vi "muPathSamplingFPGA27.vi"() -> ()   [LabVIEW 2017]
uses:
  <vilib>/rvi/Emulation/niFpgaSctlEmulationGetInTimedLoop.vi
  <vilib>/rvi/Emulation/niFpgaProcessEmulError.vi
  <vilib>/rvi/Emulation/niFpgaGetClockAttributes.vi
  <vilib>/rvi/Emulation/niFpgaEmulationReportErrorSimple.vi
  <vilib>/rvi/eio/common/nirviEmuTemplateMethod_errors.vi
  <vilib>/rvi/Emulation/niFpgaCriticalErrorInLSC.vi
  <vilib>/rvi/interface/RandomDataEmulation/niFpgaRandomDataHandleErrors.vi
  <vilib>/eio/EIONode/EIONode.xnode
  <vilib>/rvi/DataTransferAndStorage/Container/XNode/niFpgaContainer.xnode
  <vilib>/rvi/interface/RandomDataEmulation/nirviRandomDataFpgaReadWriteTemplate.vi
panel:
  in  "pixel segment":u32
  out "x output":fxp<+/-,64,29>=0.00029289722442626953
  out "x sensor":fxp<+/-,20,5>
  out "y output":fxp<+/-,64,29>=0.29396580904722214
  out "y sensor":fxp<+/-,20,5>=-0.285125732421875
  in  "XY Clock (uSec)":fxp<+,32,32>=50.0
  out "z output":fxp<+/-,64,29>=-3.5890110712498426
  out "deflection sensor":fxp<+/-,20,5>=-0.271331787109375
  in  "Z Clock (uSec)":fxp<+,32,32>=10.0
  out "ToRead":u32
  in  "Stage Clock (uSec)":fxp<+,32,32>=500.0
  in  "Sampling Clock (uSec)":fxp<+,32,32>=1500.0
  in  "muPathUpdate Clock (uSec)":fxp<+,32,32>=2400.0
  in  "initial image_x":u16=1
  in  "initial image_y":u16=1
  out "zControlMode":bool
  out "a tor buffer":fxp<+,17,1>[](array[numeric])=[1.9999847412109375, 1.9999847412109375, 1.9999847412109375, 1.9999847412109375, 1.9999847412109375, 1.9999847412109375, 1.9999847412109375, 1.9999847412109375, 1.9999847412109375, 1.9999847412109375, 1.9999847412109375, 1.9999847412109375, 1.9999847412109375, 1.9999847412109375, 1.9999847412109375, 1.9999847412109375, 1.9999847412109375, 1.9999847412109375, 1.9999847412109375, 1.9999847412109375, 1.9999847412109375, 1.9999847412109375, 1.9999847412109375, 1.9999847412109375, 1.9999847412109375]
  out "b tor buffer":fxp<+,17,1>[](array[numeric])=[1.9999847412109375, 1.9999847412109375, 1.9999847412109375, 1.9999847412109375, 1.9999847412109375, 1.9999847412109375, 1.9999847412109375, 1.9999847412109375, 1.9999847412109375, 1.9999847412109375, 1.9999847412109375, 1.9999847412109375, 1.9999847412109375, 1.9999847412109375, 1.9999847412109375, 1.9999847412109375, 1.9999847412109375, 1.9999847412109375, 1.9999847412109375, 1.9999847412109375, 1.9999847412109375, 1.9999847412109375, 1.9999847412109375, 1.9999847412109375, 1.9999847412109375]
  out "x_pos":fxp<+/-,50,5>=0.005859375
  out "y_pos":fxp<+/-,50,5>=0.005859375
  out "signalToStop":bool
  in  "deflection control":T1={"SetPoint (V)"=0.0, "scanning I"=0.03125, "scanning P"=0.0498046875, "Initial I (V)"=0.0, "Upper Limit (V)"=8.0, "Lower Limit (V)"=-8.0, "approach I"=0.03125, "approach P"=0.0498046875}
  in  "z control":T2={"SetPoint (V)"=-0.19999980926513672, "I"=0.03125, "P"=0.0498046875, "Initial I (V)"=0.0, "Upper Limit (V)"=8.0, "Lower Limit (V)"=-8.0}
  out "stageIndicator":u8=1
  in  "x threshold":fxp<+/-,20,5>=0.0050048828125
  in  "y threshold":fxp<+/-,20,5>=0.0050048828125
  in  "z threshold":fxp<+/-,20,5>=0.0050048828125
  in  "deflection threshold":fxp<+/-,20,5>=0.0050048828125
  out "length":u16
  out "direction":u16
  out "x_FinalPos":fxp<+/-,50,5>
  out "y_FinalPos":fxp<+/-,50,5>
  out "SettleCheckBuffer":u16=25
  in  "y control":T3={"SetPoint (V)"=0.0, "scanning I"=0.03125, "scanning P"=0.0498046875, "Initial I (V)"=0.0, "Upper Limit (V)"=8.0, "Lower Limit (V)"=-8.0, "move I"=0.03125, "move P"=0.0302734375}
  in  "x control":T3={"SetPoint (V)"=0.0, "scanning I"=0.03125, "scanning P"=0.0498046875, "Initial I (V)"=0.0, "Upper Limit (V)"=8.0, "Lower Limit (V)"=-8.0, "move I"=0.03125, "move P"=0.0498046875}
  out "signalToInitialStageStop":bool
  out "mupathfinishSignal":bool
  in  "ImageToSample":T4={"image size_x"=256, "image size_y"=256, "sample start_x"=0.0, "sample start_y"=0.0, "sample end_x"=3.0, "sample end_y"=3.0}
  out "increment_x":fxp<+/-,50,5>=0.01171875
  out "increment_y":fxp<+/-,50,5>=0.01171875
  out "x_image_pos":u16
  out "y_image_pos":u16
  in  "x_scan threshold":fxp<+/-,20,5>=0.0050048828125
  in  "y_scan threshold":fxp<+/-,20,5>=0.0050048828125
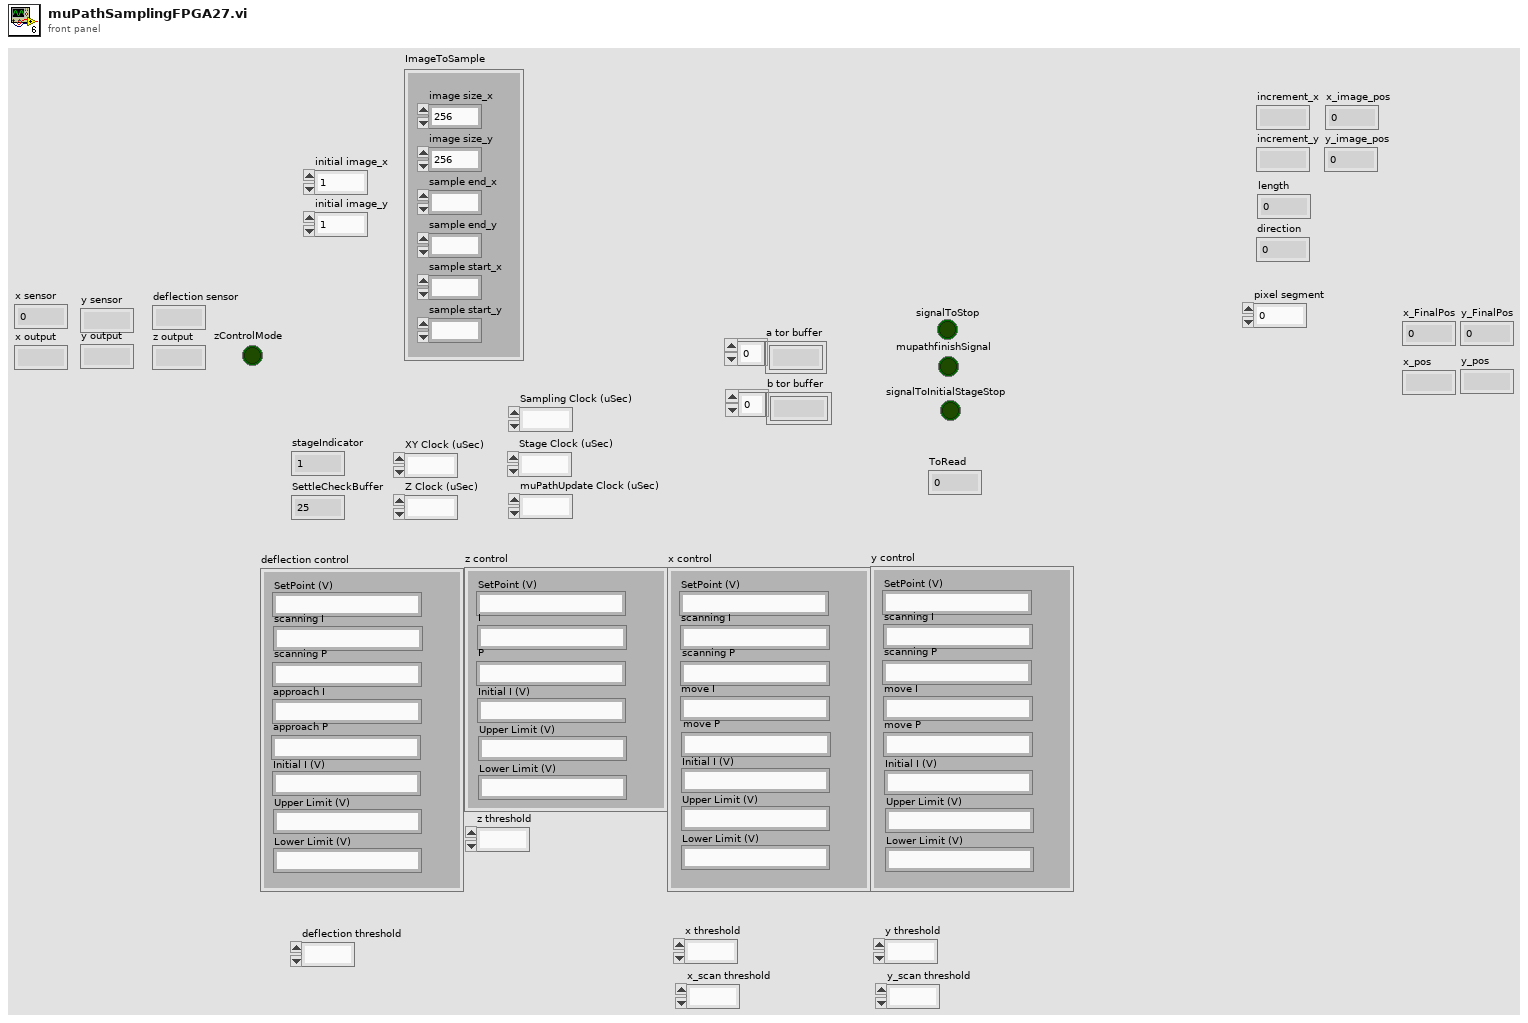
[diagram p1: front panel]
types:
  T1 = cluster{"SetPoint (V)":fxp<+/-,26,5>, "scanning I":fxp<+,21,13>, "scanning P":fxp<+,15,5>, "Initial I (V)":fxp<+/-,10,5>, "Upper Limit (V)":fxp<+/-,26,5>, "Lower Limit (V)":fxp<+/-,26,5>, "approach I":fxp<+,21,13>, "approach P":fxp<+,15,5>}
  T2 = cluster{"SetPoint (V)":fxp<+/-,26,5>, "I":fxp<+,21,13>, "P":fxp<+,15,5>, "Initial I (V)":fxp<+/-,10,5>, "Upper Limit (V)":fxp<+/-,26,5>, "Lower Limit (V)":fxp<+/-,26,5>}
  T3 = cluster{"SetPoint (V)":fxp<+/-,26,5>, "scanning I":fxp<+,21,13>, "scanning P":fxp<+,15,5>, "Initial I (V)":fxp<+/-,10,5>, "Upper Limit (V)":fxp<+/-,26,5>, "Lower Limit (V)":fxp<+/-,26,5>, "move I":fxp<+,21,13>, "move P":fxp<+,15,5>}
  T4 = cluster{"image size_x":u16, "image size_y":u16, "sample start_x":fxp<+/-,26,5>, "sample start_y":fxp<+/-,26,5>, "sample end_x":fxp<+/-,26,5>, "sample end_y":fxp<+/-,26,5>}
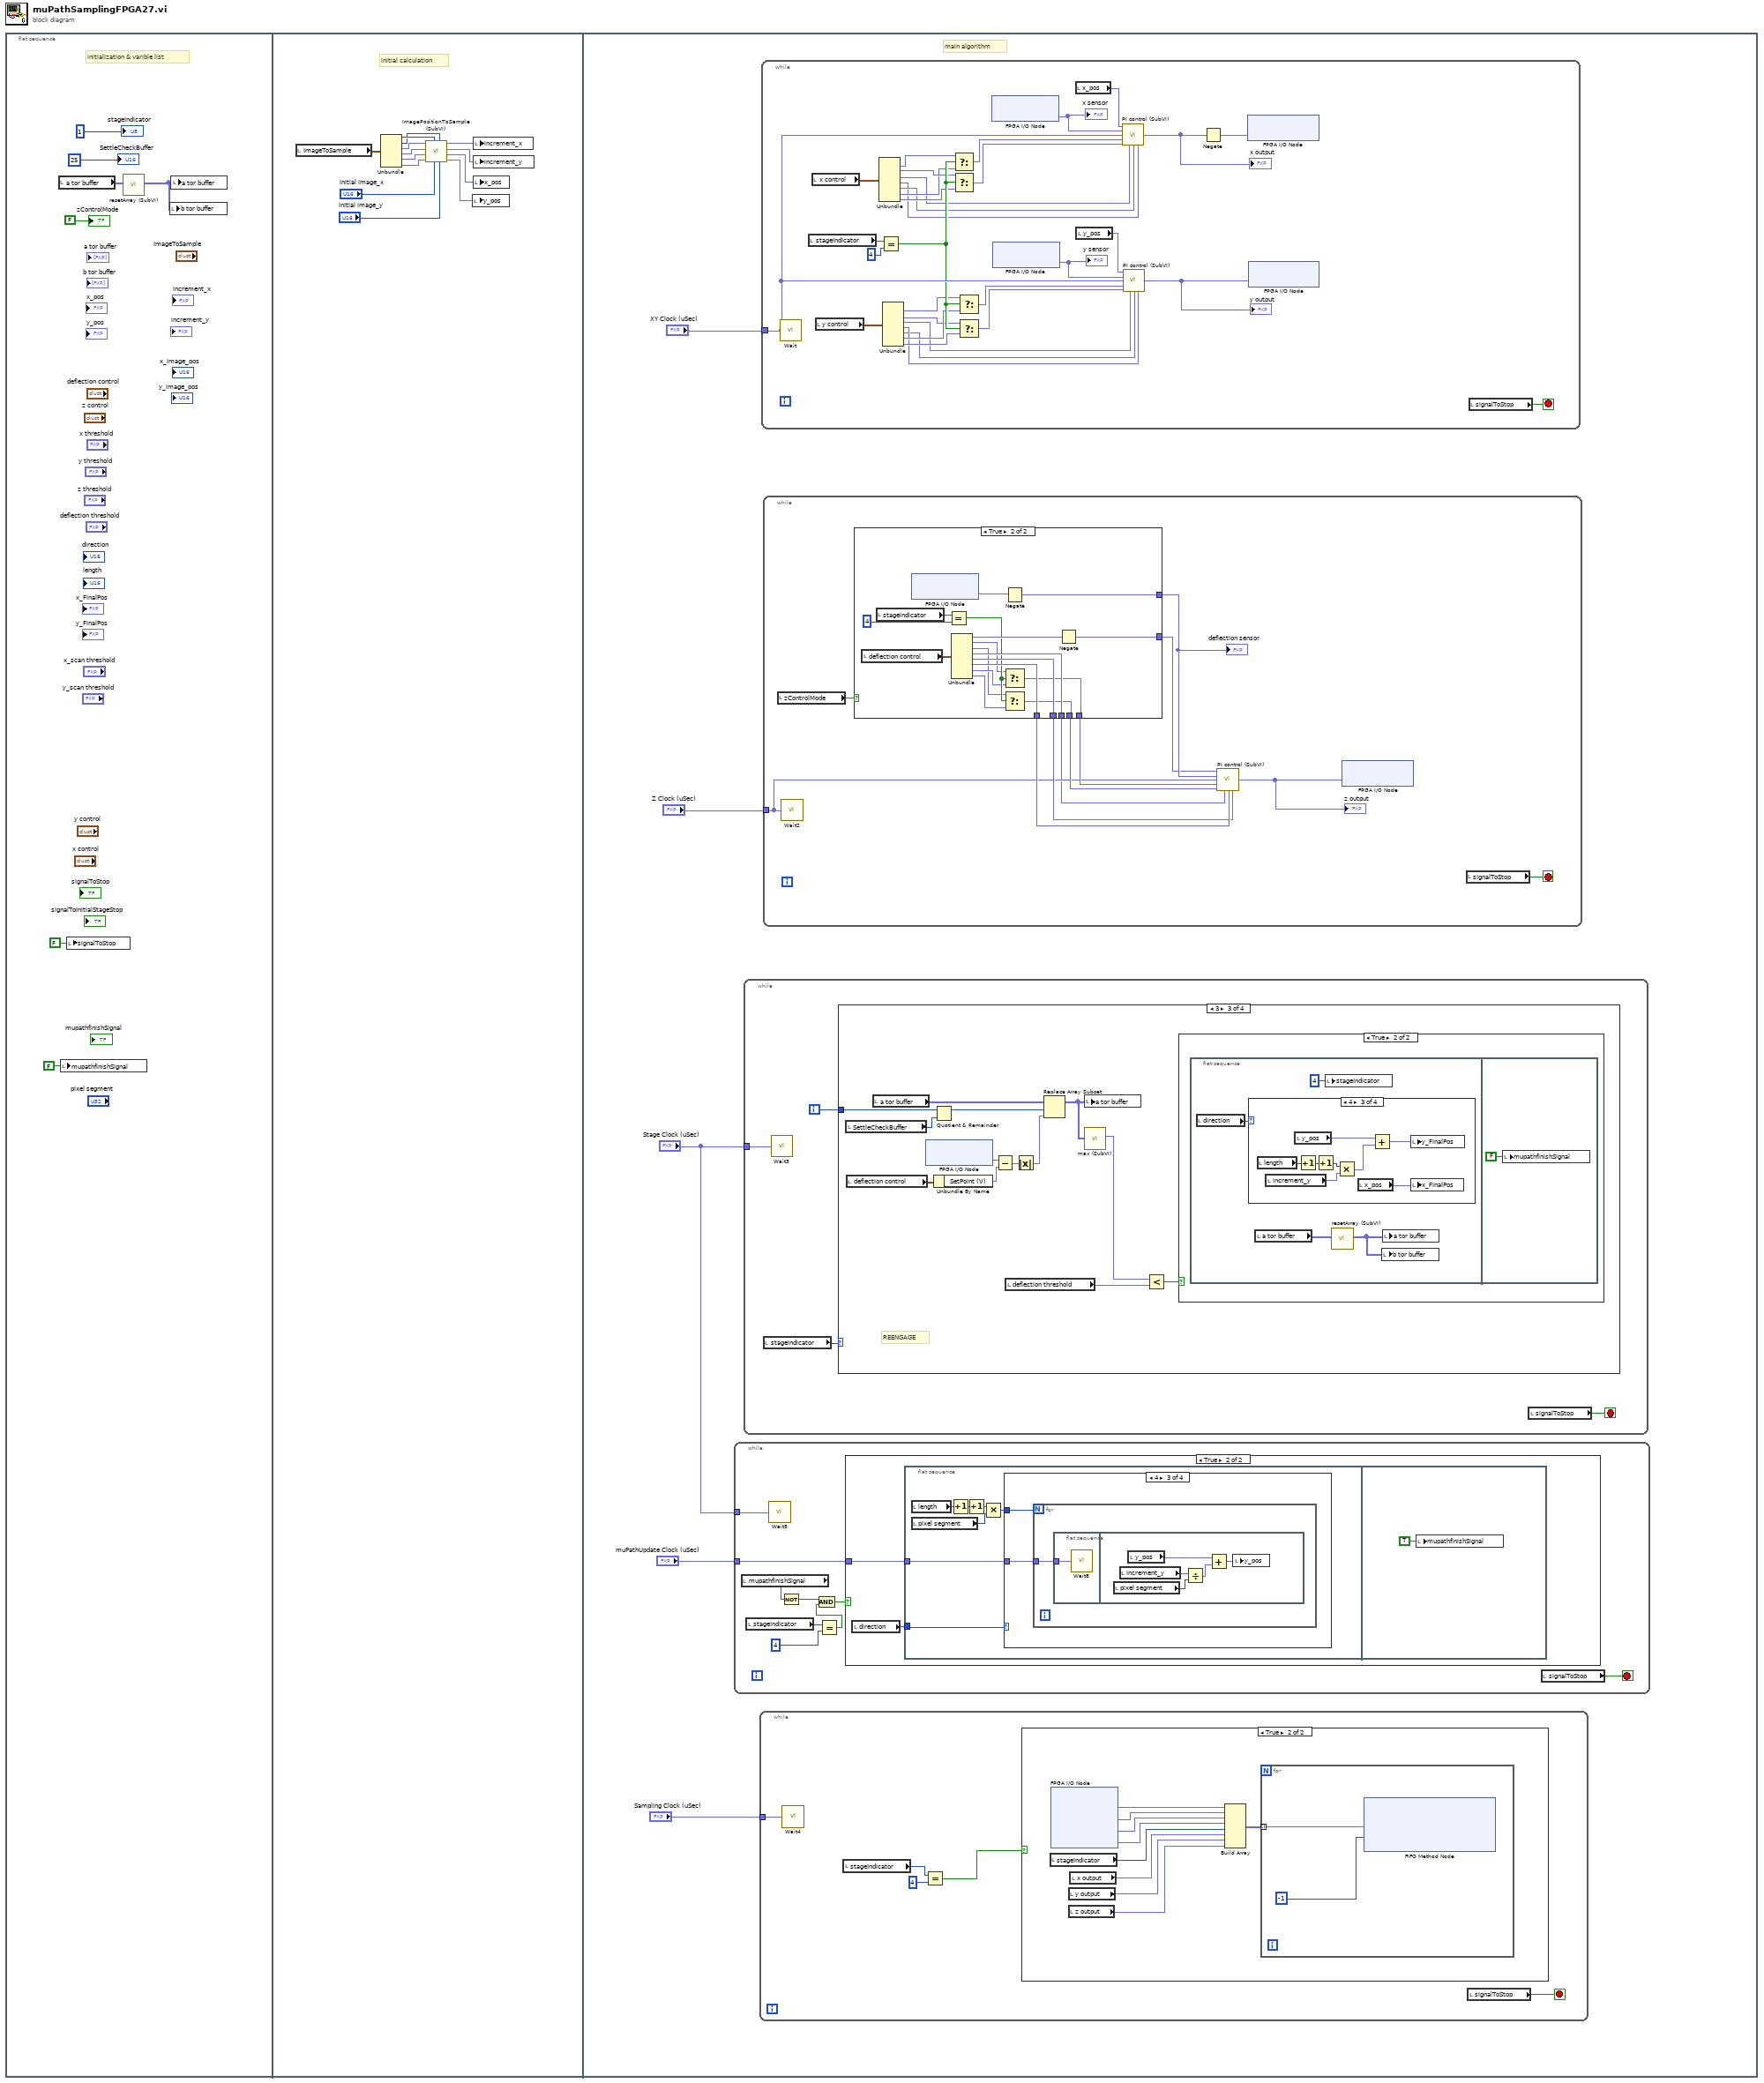
[diagram p0: block diagram]
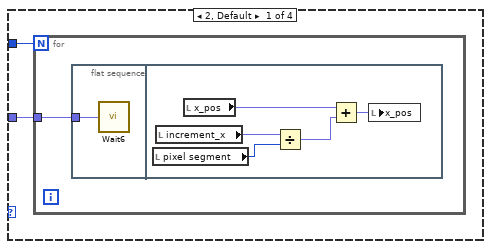
[diagram p3: hidden frame]
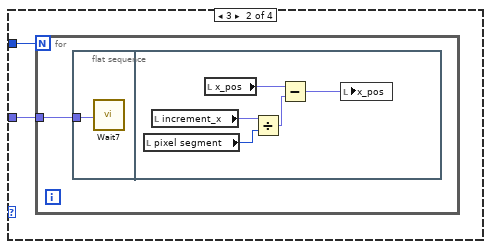
[diagram p4: hidden frame]
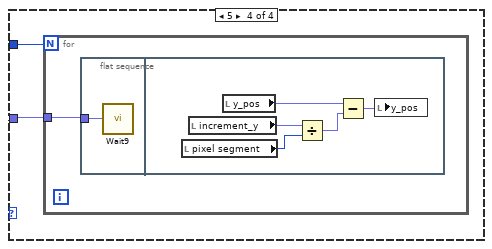
[diagram p5: hidden frame]
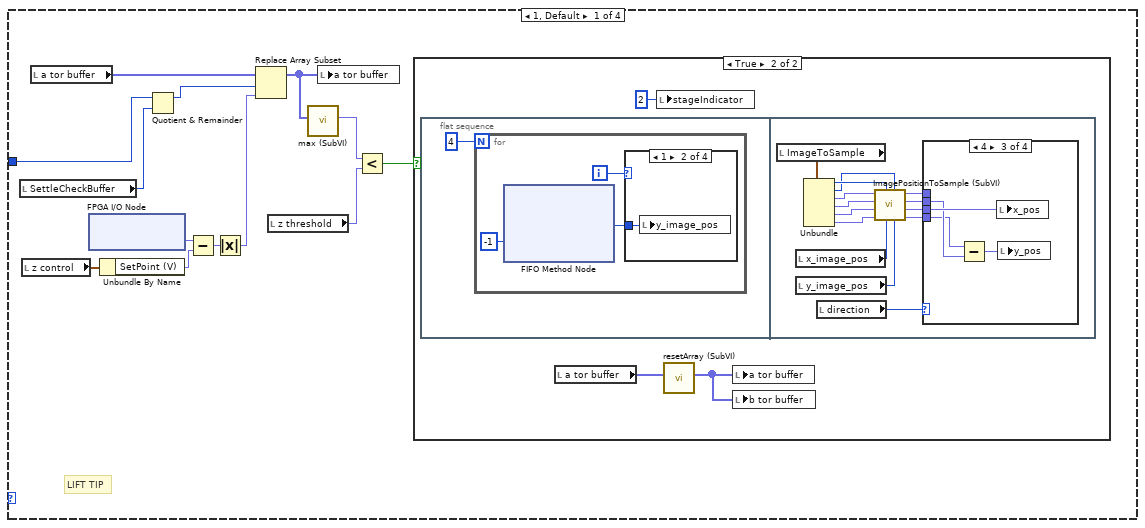
[diagram p7: hidden frame]
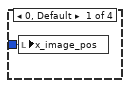
[diagram p9: hidden frame]
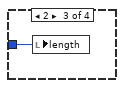
[diagram p10: hidden frame]
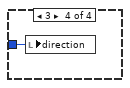
[diagram p11: hidden frame]
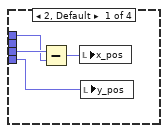
[diagram p12: hidden frame]
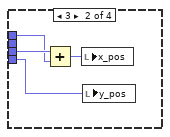
[diagram p13: hidden frame]
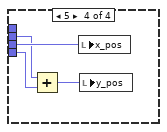
[diagram p14: hidden frame]
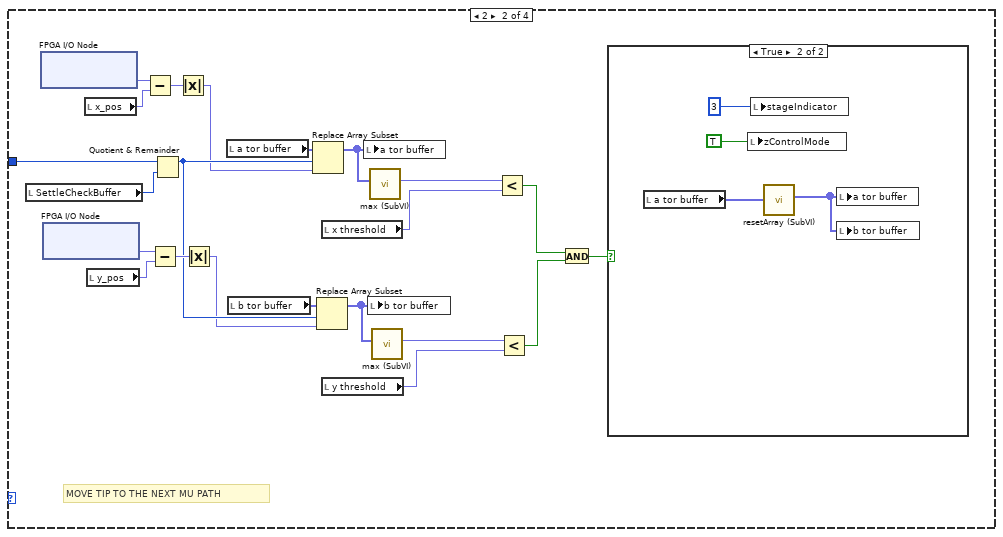
[diagram p15: hidden frame]
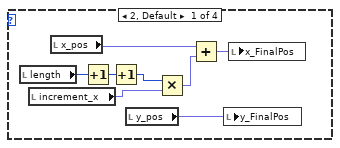
[diagram p18: hidden frame]
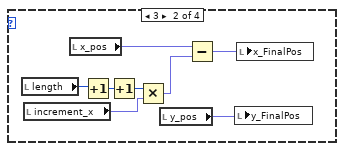
[diagram p19: hidden frame]
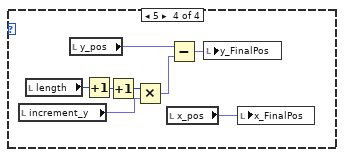
[diagram p20: hidden frame]
diagram:
  n1 = flat-sequence {
    frame #0 {
      # "initialization & varible list"
      n2 = local read "a tor buffer"() -> (w6:fxp<+,17,1>[])
      n3 = local write "mupathfinishSignal"(FALSE ("mupathfinishSignal")) -> ()
      n4 = local write "signalToStop"(FALSE ("signalToStop")) -> ()
      n5 = call "resetArray (SubVI).vi"("a samples in"=w6) -> ("a samples out"=w7:fxp<+/-,64,32>[])  [unwired: 10 in]
      n6 = local write "b tor buffer"(w7) -> ()
      n7 = local write "a tor buffer"(w7) -> ()
      "zControlMode" <- FALSE ("zControlMode")
      "stageIndicator" <- u8 1 ("stageIndicator")
      "SettleCheckBuffer" <- u16 25 ("SettleCheckLen")
    }
    frame #1 {
      # "initial calculation"
      n8 = local read "ImageToSample"() -> (w20:T4)
      n9 = Unbundle(w20) -> ("image size_x"=w19:u16, "image size_y"=w18:u16, "sample start_x"=w17:fxp<+/-,26,5>, "sample start_y"=w16:fxp<+/-,26,5>, "sample end_x"=w15:fxp<+/-,26,5>, "sample end_y"=w14:fxp<+/-,26,5>)
      n10 = call "ImagePositionToSample (SubVI).vi"("image_y"="initial image_y", "image size_y"=w18, "image_x"="initial image_x", "image size_x"=w19, "sample end_y"=w14, "sample end_x"=w15, "sample start_y"=w16, "sample start_x"=w17) -> ("sample_y"=w8:fxp<+/-,26,5>, "sample_x"=w9:fxp<+/-,26,5>, "increment_y"=w10:fxp<+/-,26,5>, "increment_x"=w11:fxp<+/-,26,5>)
      n11 = local write "y_pos"(w8) -> ()
      n12 = local write "increment_x"(w11) -> ()
      n13 = local write "increment_y"(w10) -> ()
      n14 = local write "x_pos"(w9) -> ()
    }
    frame #2 {
      # "main algorithm"
      n15 = while {
        tunnel: "Stage Clock (uSec)" -> [w33]
        tunnel: "muPathUpdate Clock (uSec)" -> [w30]
        stop <- w34 stop-if-true
        n16 = local read "mupathfinishSignal"() -> (w27:bool)
        n17 = local read "stageIndicator"() -> (w32:u8)
        n18 = call "Wait5"("Count(uSec)"=w33) -> ()  [unwired: 1 out]
        n19 = Not(x=w27) -> (.not. x?=w26:bool)
        n20 = Equal?(x=w32, y=u8 4) -> (x = y?=w29:bool)
        n21 = And(x=w26, y=w29) -> (x .and. y?=w28:bool)
        n22 = case shown="True" w28 {
          tunnel: w30 -> [_ w36]
          frame False {
          }
          frame True {
            n23 = local read "direction"() -> (w35:u16)
            n24 = flat-sequence {
              tunnel: w36 -> [w43]
              tunnel: w35 -> [w42]
              frame #0 {
                n25 = local read "length"() -> (w41:u16)
                n26 = local read "pixel segment"() -> (w39:u32)
                n27 = Increment(x=w41) -> (x+1=w38:u16)
                n28 = Increment(x=w38) -> (x+1=w37:u16)
                n29 = Multiply(x=w37, y=w39) -> (x*y=w40:u32)
                n30 = case shown="4" w42 {
                  tunnel: w43 -> [w45 w54 w63 w72]
                  tunnel: w40 -> [w44 w53 w62 w71]
                  frame 2, Default {
                    n31 = for {
                      N: w44 -> [_]
                      tunnel: w45 -> [w46]
                      n32 = flat-sequence {
                        tunnel: w46 -> [w47]
                        frame #0 {
                          n33 = call "Wait6"("Count(uSec)"=w47) -> ()  [unwired: 1 out]
                        }
                        frame #1 {
                          n34 = local read "pixel segment"() -> (w48:u32)
                          n35 = local read "increment_x"() -> (w50:fxp<+/-,50,5>)
                          n36 = local read "x_pos"() -> (w52:fxp<+/-,50,5>)
                          n37 = Divide(x=w50, y=w48) -> (x/y=w49:fxp<+/-,64,5>)
                          n38 = Add(x=w52, y=w49) -> (x+y=w51:fxp<+/-,64,6>)
                          n39 = local write "x_pos"(w51) -> ()
                        }
                      }
                    }
                  }
                  frame 3 {
                    n40 = for {
                      N: w53 -> [_]
                      tunnel: w54 -> [w55]
                      n41 = flat-sequence {
                        tunnel: w55 -> [w56]
                        frame #0 {
                          n42 = call "Wait7"("Count(uSec)"=w56) -> ()  [unwired: 1 out]
                        }
                        frame #1 {
                          n43 = local read "pixel segment"() -> (w57:u32)
                          n44 = local read "increment_x"() -> (w59:fxp<+/-,50,5>)
                          n45 = local read "x_pos"() -> (w61:fxp<+/-,50,5>)
                          n46 = Divide(x=w59, y=w57) -> (x/y=w58:fxp<+/-,64,5>)
                          n47 = Subtract(x=w61, y=w58) -> (x-y=w60:fxp<+/-,64,6>)
                          n48 = local write "x_pos"(w60) -> ()
                        }
                      }
                    }
                  }
                  frame 4 {
                    n49 = for {
                      N: w62 -> [_]
                      tunnel: w63 -> [w64]
                      n50 = flat-sequence {
                        tunnel: w64 -> [w65]
                        frame #0 {
                          n51 = call "Wait8"("Count(uSec)"=w65) -> ()  [unwired: 1 out]
                        }
                        frame #1 {
                          n52 = local read "pixel segment"() -> (w66:u32)
                          n53 = local read "increment_y"() -> (w68:fxp<+/-,50,5>)
                          n54 = local read "y_pos"() -> (w70:fxp<+/-,50,5>)
                          n55 = Divide(x=w68, y=w66) -> (x/y=w67:fxp<+/-,64,5>)
                          n56 = Add(x=w70, y=w67) -> (x+y=w69:fxp<+/-,64,6>)
                          n57 = local write "y_pos"(w69) -> ()
                        }
                      }
                    }
                  }
                  frame 5 {
                    n58 = for {
                      N: w71 -> [_]
                      tunnel: w72 -> [w73]
                      n59 = flat-sequence {
                        tunnel: w73 -> [w74]
                        frame #0 {
                          n60 = call "Wait9"("Count(uSec)"=w74) -> ()  [unwired: 1 out]
                        }
                        frame #1 {
                          n61 = local read "pixel segment"() -> (w76:u32)
                          n62 = local read "increment_y"() -> (w77:fxp<+/-,50,5>)
                          n63 = local read "y_pos"() -> (w79:fxp<+/-,50,5>)
                          n64 = Divide(x=w77, y=w76) -> (x/y=w75:fxp<+/-,64,5>)
                          n65 = Subtract(x=w79, y=w75) -> (x-y=w78:fxp<+/-,64,6>)
                          n66 = local write "y_pos"(w78) -> ()
                        }
                      }
                    }
                  }
                }
              }
              frame #1 {
                n67 = local write "mupathfinishSignal"(TRUE ("mupathfinishSignal")) -> ()
              }
            }
          }
        }
        n68 = local read "signalToStop"() -> (w34:bool)
      }
      n69 = while {
        tunnel: "Stage Clock (uSec)" -> [w98]
        i -> [w97]
        stop <- w100 stop-if-true
        n70 = local read "stageIndicator"() -> (w99:u8)
        n71 = call "Wait3"("Count(uSec)"=w98) -> ()  [unwired: 1 out]
        n72 = case shown="3" w99 {
          tunnel: w97 -> [w112 w169 w189 w248]
          frame 1, Default {
            # "LIFT TIP"
            n73 = local read "SettleCheckBuffer"() -> (w111:u16)
            n74 = local read "z control"() -> (w107:T2)
            n75 = local read "a tor buffer"() -> (w110:fxp<+,17,1>[])
            n76 = xnode "FPGA I/O Node"() -> ("Mod1/AI2"=w108:fxp<+/-,20,5>)  [unwired: 1 in, 1 out]
            n77 = Unbundle By Name(w107) -> ("SetPoint (V)"=w106:fxp<+/-,26,5>)
            n78 = Quotient & Remainder(x=w112, y=w111) -> (x-y*floor(x/y)=w105:i32)  [unwired: 1 out]
            n79 = Subtract(x=w108, y=w106) -> (x-y=w109:fxp<+/-,27,6>)
            n80 = Absolute Value(x=w109) -> (abs(x)=w104:fxp<+,26,5>)
            n81 = Replace Array Subset(array=w110, new element=w104, index=w105) -> (w102:fxp<+,17,1>[])
            n82 = local read "z threshold"() -> (w103:fxp<+/-,20,5>)
            n83 = call "max (SubVI).vi"("initialized array"=w102) -> ("y"=w101:fxp<+/-,64,32>)  [unwired: 10 in]
            n84 = local write "a tor buffer"(w102) -> ()
            n85 = Less?(x=w101, y=w103) -> (x < y?=w113:bool)
            n86 = case shown="True" w113 {
              frame False {
              }
              frame True {
                n87 = flat-sequence {
                  frame #0 {
                    n88 = for {
                      N: 4 -> [_]
                      i -> [w120]
                      n89 = xnode ("FIFO Method Node")("Timeout"=-1) -> ("Element"=w118:u16)  [unwired: 1 in, 2 out]
                      n90 = case shown="1" w120 {
                        tunnel: w118 -> [w121 w122 w123 w124]
                        frame 0, Default {
                          n91 = local write "x_image_pos"(w121) -> ()
                        }
                        frame 1 {
                          n92 = local write "y_image_pos"(w122) -> ()
                        }
                        frame 2 {
                          n93 = local write "length"(w123) -> ()
                        }
                        frame 3 {
                          n94 = local write "direction"(w124) -> ()
                        }
                      }
                    }
                  }
                  frame #1 {
                    n95 = local read "ImageToSample"() -> (w138:T4)
                    n96 = local read "x_image_pos"() -> (w131:u16)
                    n97 = local read "y_image_pos"() -> (w130:u16)
                    n98 = Unbundle(w138) -> ("image size_x"=w137:u16, "image size_y"=w136:u16, "sample start_x"=w135:fxp<+/-,26,5>, "sample start_y"=w134:fxp<+/-,26,5>, "sample end_x"=w133:fxp<+/-,26,5>, "sample end_y"=w132:fxp<+/-,26,5>)
                    n99 = local read "direction"() -> (w129:u16)
                    n100 = call "ImagePositionToSample (SubVI).vi"("image_y"=w130, "image size_y"=w136, "image_x"=w131, "image size_x"=w137, "sample end_y"=w132, "sample end_x"=w133, "sample start_y"=w134, "sample start_x"=w135) -> ("sample_y"=w128:fxp<+/-,26,5>, "sample_x"=w127:fxp<+/-,26,5>, "increment_y"=w125:fxp<+/-,26,5>, "increment_x"=w126:fxp<+/-,26,5>)
                    n101 = case shown="4" w129 {
                      tunnel: w128 -> [w142 w146 w147 w152]
                      tunnel: w127 -> [w141 w145 w150 w154]
                      tunnel: w126 -> [w140 w144 _ _]
                      tunnel: w125 -> [_ _ w148 w153]
                      frame 2, Default {
                        n102 = Subtract(x=w141, y=w140) -> (x-y=w139:fxp<+/-,27,6>)
                        n103 = local write "x_pos"(w139) -> ()
                        n104 = local write "y_pos"(w142) -> ()
                      }
                      frame 3 {
                        n105 = Add(x=w145, y=w144) -> (x+y=w143:fxp<+/-,27,6>)
                        n106 = local write "x_pos"(w143) -> ()
                        n107 = local write "y_pos"(w146) -> ()
                      }
                      frame 4 {
                        n108 = Subtract(x=w147, y=w148) -> (x-y=w149:fxp<+/-,27,6>)
                        n109 = local write "x_pos"(w150) -> ()
                        n110 = local write "y_pos"(w149) -> ()
                      }
                      frame 5 {
                        n111 = Add(x=w153, y=w152) -> (x+y=w151:fxp<+/-,27,6>)
                        n112 = local write "x_pos"(w154) -> ()
                        n113 = local write "y_pos"(w151) -> ()
                      }
                    }
                  }
                }
                n114 = local read "a tor buffer"() -> (w115:fxp<+,17,1>[])
                n115 = local write "stageIndicator"(u8 2 ("stageIndicator")) -> ()
                n116 = call "resetArray (SubVI).vi"("a samples in"=w115) -> ("a samples out"=w114:fxp<+/-,64,32>[])  [unwired: 10 in]
                n117 = local write "a tor buffer"(w114) -> ()
                n118 = local write "b tor buffer"(w114) -> ()
              }
            }
          }
          frame 2 {
            # "MOVE TIP TO THE NEXT MU PATH"
            n119 = local read "SettleCheckBuffer"() -> (w168:u16)
            n120 = xnode "FPGA I/O Node"() -> ("Mod1/AI0"=w175:fxp<+/-,20,5>)  [unwired: 1 in, 1 out]
            n121 = xnode "FPGA I/O Node"() -> ("Mod1/AI1"=w173:fxp<+/-,20,5>)  [unwired: 1 in, 1 out]
            n122 = local read "x_pos"() -> (w172:fxp<+/-,50,5>)
            n123 = local read "y_pos"() -> (w171:fxp<+/-,50,5>)
            n124 = Subtract(x=w175, y=w172) -> (x-y=w176:fxp<+/-,51,6>)
            n125 = Subtract(x=w173, y=w171) -> (x-y=w174:fxp<+/-,51,6>)
            n126 = Quotient & Remainder(x=w169, y=w168) -> (x-y*floor(x/y)=w166:i32)  [unwired: 1 out]
            n127 = Absolute Value(x=w176) -> (abs(x)=w164:fxp<+,50,5>)
            n128 = Absolute Value(x=w174) -> (abs(x)=w163:fxp<+,50,5>)
            n129 = local read "a tor buffer"() -> (w167:fxp<+,17,1>[])
            n130 = local read "b tor buffer"() -> (w165:fxp<+,17,1>[])
            n131 = Replace Array Subset(array=w167, new element=w164, index=w166) -> (w157:fxp<+,17,1>[])
            n132 = Replace Array Subset(array=w165, new element=w163, index=w166) -> (w155:fxp<+,17,1>[])
            n133 = local read "x threshold"() -> (w162:fxp<+/-,20,5>)
            n134 = local read "y threshold"() -> (w161:fxp<+/-,20,5>)
            n135 = local write "a tor buffer"(w157) -> ()
            n136 = local write "b tor buffer"(w155) -> ()
            n137 = call "max (SubVI).vi"("initialized array"=w157) -> ("y"=w158:fxp<+/-,64,32>)  [unwired: 10 in]
            n138 = call "max (SubVI).vi"("initialized array"=w155) -> ("y"=w156:fxp<+/-,64,32>)  [unwired: 10 in]
            n139 = Less?(x=w158, y=w162) -> (x < y?=w160:bool)
            n140 = Less?(x=w156, y=w161) -> (x < y?=w159:bool)
            n141 = And(x=w160, y=w159) -> (x .and. y?=w170:bool)
            n142 = case shown="True" w170 {
              frame False {
              }
              frame True {
                n143 = local read "a tor buffer"() -> (w178:fxp<+,17,1>[])
                n144 = local write "zControlMode"(TRUE ("signalToStop")) -> ()
                n145 = local write "stageIndicator"(u8 3 ("stageIndicator")) -> ()
                n146 = call "resetArray (SubVI).vi"("a samples in"=w178) -> ("a samples out"=w177:fxp<+/-,64,32>[])  [unwired: 10 in]
                n147 = local write "a tor buffer"(w177) -> ()
                n148 = local write "b tor buffer"(w177) -> ()
              }
            }
          }
          frame 3 {
            # "REENGAGE"
            n149 = local read "SettleCheckBuffer"() -> (w188:u16)
            n150 = local read "deflection control"() -> (w191:T1)
            n151 = local read "a tor buffer"() -> (w186:fxp<+,17,1>[])
            n152 = xnode "FPGA I/O Node"() -> ("Mod1/AI3"=w192:fxp<+/-,20,5>)  [unwired: 1 in, 1 out]
            n153 = Quotient & Remainder(x=w189, y=w188) -> (x-y*floor(x/y)=w187:i32)  [unwired: 1 out]
            n154 = Unbundle By Name(w191) -> ("SetPoint (V)"=w190:fxp<+/-,26,5>)
            n155 = Subtract(x=w192, y=w190) -> (x-y=w193:fxp<+/-,27,6>)
            n156 = local read "deflection threshold"() -> (w183:fxp<+/-,20,5>)
            n157 = Absolute Value(x=w193) -> (abs(x)=w185:fxp<+,26,5>)
            n158 = Replace Array Subset(array=w186, new element=w185, index=w187) -> (w182:fxp<+,17,1>[])
            n159 = local write "a tor buffer"(w182) -> ()
            n160 = call "max (SubVI).vi"("initialized array"=w182) -> ("y"=w181:fxp<+/-,64,32>)  [unwired: 10 in]
            n161 = Less?(x=w181, y=w183) -> (x < y?=w184:bool)
            n162 = case shown="True" w184 {
              frame False {
              }
              frame True {
                n163 = flat-sequence {
                  frame #0 {
                    n164 = local read "direction"() -> (w196:u16)
                    n165 = case shown="4" w196 {
                      frame 2, Default {
                        n166 = local read "length"() -> (w198:u16)
                        n167 = local read "increment_x"() -> (w203:fxp<+/-,50,5>)
                        n168 = local read "x_pos"() -> (w205:fxp<+/-,50,5>)
                        n169 = Increment(x=w198) -> (x+1=w199:u16)
                        n170 = Increment(x=w199) -> (x+1=w200:u16)
                        n171 = local read "y_pos"() -> (w201:fxp<+/-,50,5>)
                        n172 = Multiply(x=w200, y=w203) -> (x*y=w202:fxp<+/-,64,21>)
                        n173 = Add(x=w205, y=w202) -> (x+y=w204:fxp<+/-,64,22>)
                        n174 = local write "y_FinalPos"(w201) -> ()
                        n175 = local write "x_FinalPos"(w204) -> ()
                      }
                      frame 3 {
                        n176 = local read "length"() -> (w208:u16)
                        n177 = local read "increment_x"() -> (w211:fxp<+/-,50,5>)
                        n178 = local read "x_pos"() -> (w213:fxp<+/-,50,5>)
                        n179 = Increment(x=w208) -> (x+1=w207:u16)
                        n180 = Increment(x=w207) -> (x+1=w206:u16)
                        n181 = Multiply(x=w206, y=w211) -> (x*y=w210:fxp<+/-,64,21>)
                        n182 = local read "y_pos"() -> (w209:fxp<+/-,50,5>)
                        n183 = Subtract(x=w213, y=w210) -> (x-y=w212:fxp<+/-,64,22>)
                        n184 = local write "y_FinalPos"(w209) -> ()
                        n185 = local write "x_FinalPos"(w212) -> ()
                      }
                      frame 4 {
                        n186 = local read "length"() -> (w216:u16)
                        n187 = local read "increment_y"() -> (w219:fxp<+/-,50,5>)
                        n188 = local read "y_pos"() -> (w221:fxp<+/-,50,5>)
                        n189 = Increment(x=w216) -> (x+1=w215:u16)
                        n190 = Increment(x=w215) -> (x+1=w214:u16)
                        n191 = Multiply(x=w214, y=w219) -> (x*y=w218:fxp<+/-,64,21>)
                        n192 = local read "x_pos"() -> (w217:fxp<+/-,50,5>)
                        n193 = Add(x=w221, y=w218) -> (x+y=w220:fxp<+/-,64,22>)
                        n194 = local write "y_FinalPos"(w220) -> ()
                        n195 = local write "x_FinalPos"(w217) -> ()
                      }
                      frame 5 {
                        n196 = local read "increment_y"() -> (w226:fxp<+/-,50,5>)
                        n197 = local read "length"() -> (w224:u16)
                        n198 = local read "y_pos"() -> (w229:fxp<+/-,50,5>)
                        n199 = Increment(x=w224) -> (x+1=w223:u16)
                        n200 = Increment(x=w223) -> (x+1=w222:u16)
                        n201 = Multiply(x=w222, y=w226) -> (x*y=w227:fxp<+/-,64,21>)
                        n202 = local read "x_pos"() -> (w225:fxp<+/-,50,5>)
                        n203 = Subtract(x=w229, y=w227) -> (x-y=w228:fxp<+/-,64,22>)
                        n204 = local write "y_FinalPos"(w228) -> ()
                        n205 = local write "x_FinalPos"(w225) -> ()
                      }
                    }
                    n206 = local read "a tor buffer"() -> (w195:fxp<+,17,1>[])
                    n207 = local write "stageIndicator"(u8 4 ("stageIndicator")) -> ()
                    n208 = call "resetArray (SubVI).vi"("a samples in"=w195) -> ("a samples out"=w194:fxp<+/-,64,32>[])  [unwired: 10 in]
                    n209 = local write "b tor buffer"(w194) -> ()
                    n210 = local write "a tor buffer"(w194) -> ()
                  }
                  frame #1 {
                    n211 = local write "mupathfinishSignal"(FALSE ("mupathfinishSignal")) -> ()
                  }
                }
              }
            }
          }
          frame 4 {
            # "SCAN"
            n212 = local read "SettleCheckBuffer"() -> (w247:u16)
            n213 = xnode "FPGA I/O Node"() -> ("Mod1/AI1"=w252:fxp<+/-,20,5>)  [unwired: 1 in, 1 out]
            n214 = xnode "FPGA I/O Node"() -> ("Mod1/AI0"=w254:fxp<+/-,20,5>)  [unwired: 1 in, 1 out]
            n215 = local read "y_FinalPos"() -> (w249:fxp<+/-,50,5>)
            n216 = local read "x_FinalPos"() -> (w250:fxp<+/-,50,5>)
            n217 = Subtract(x=w252, y=w249) -> (x-y=w251:fxp<+/-,51,6>)
            n218 = Subtract(x=w254, y=w250) -> (x-y=w253:fxp<+/-,51,6>)
            n219 = Quotient & Remainder(x=w248, y=w247) -> (x-y*floor(x/y)=w246:i32)  [unwired: 1 out]
            n220 = Absolute Value(x=w251) -> (abs(x)=w245:fxp<+,50,5>)
            n221 = Absolute Value(x=w253) -> (abs(x)=w244:fxp<+,50,5>)
            n222 = local read "b tor buffer"() -> (w242:fxp<+,17,1>[])
            n223 = local read "a tor buffer"() -> (w243:fxp<+,17,1>[])
            n224 = local read "x_scan threshold"() -> (w241:fxp<+/-,20,5>)
            n225 = local read "y_scan threshold"() -> (w240:fxp<+/-,20,5>)
            n226 = Replace Array Subset(array=w243, new element=w244, index=w246) -> (w234:fxp<+,17,1>[])
            n227 = Replace Array Subset(array=w242, new element=w245, index=w246) -> (w237:fxp<+,17,1>[])
            n228 = local read "mupathfinishSignal"() -> (w231:bool)
            n229 = local write "a tor buffer"(w234) -> ()
            n230 = call "max (SubVI).vi"("initialized array"=w234) -> ("y"=w235:fxp<+/-,64,32>)  [unwired: 10 in]
            n231 = local write "b tor buffer"(w237) -> ()
            n232 = call "max (SubVI).vi"("initialized array"=w237) -> ("y"=w236:fxp<+/-,64,32>)  [unwired: 10 in]
            n233 = Less?(x=w235, y=w241) -> (x < y?=w239:bool)
            n234 = Less?(x=w236, y=w240) -> (x < y?=w238:bool)
            n235 = And(x=w239, y=w238) -> (x .and. y?=w232:bool)
            n236 = And(x=w232, y=w231) -> (x .and. y?=w233:bool)
            n237 = case shown="True" w233 {
              frame False {
              }
              frame True {
                n238 = xnode ("FIFO Method Node")() -> ("Number of Elements to Read"=w259:u32)  [unwired: 1 in, 1 out]
                "ToRead" <- w259
                n239 = local read "a tor buffer"() -> (w256:fxp<+,17,1>[])
                n240 = flat-sequence {
                  frame #0 {
                    n241 = local write "stageIndicator"(u8 1 ("stageIndicator")) -> ()
                  }
                  frame #1 {
                    n242 = local write "mupathfinishSignal"(FALSE ("mupathfinishSignal")) -> ()
                  }
                }
                n243 = local write "zControlMode"(FALSE ("zControlMode")) -> ()
                n244 = call "resetArray (SubVI).vi"("a samples in"=w256) -> ("a samples out"=w255:fxp<+/-,64,32>[])  [unwired: 10 in]
                n245 = local write "b tor buffer"(w255) -> ()
                n246 = local write "a tor buffer"(w255) -> ()
                n247 = Less Or Equal?(x=w259, y=u32 0) -> (x <= y?=w257:bool)
                n248 = local write "signalToStop"(w257) -> ()
              }
            }
          }
        }
        n249 = local read "signalToStop"() -> (w100:bool)
      }
      n250 = while {
        tunnel: "Sampling Clock (uSec)" -> [w85]
        stop <- w84 stop-if-true
        n251 = call "Wait4"("Count(uSec)"=w85) -> ()  [unwired: 1 out]
        n252 = local read "stageIndicator"() -> (w82:u8)
        n253 = Equal?(x=w82, y=u8 4) -> (x = y?=w83:bool)
        n254 = case shown="True" w83 {
          frame False {
          }
          frame True {
            n255 = local read "stageIndicator"() -> (w89:u8)
            n256 = xnode "FPGA I/O Node"() -> ("Mod1/AI0"=w93:fxp<+/-,20,5>, "Mod1/AI1"=w92:fxp<+/-,20,5>, "Mod1/AI2"=w91:fxp<+/-,20,5>, "Mod1/AI3"=w90:fxp<+/-,20,5>)  [unwired: 4 in, 4 out]
            n257 = local read "y output"() -> (w87:fxp<+/-,64,29>)
            n258 = local read "z output"() -> (w86:fxp<+/-,64,29>)
            n259 = local read "x output"() -> (w88:fxp<+/-,64,29>)
            n260 = Build Array(w93, w92, w91, w90, w89, w88, w87, w86) -> (w94:fxp<+/-,64,29>[])
            n261 = for {
              tunnel: w94 -> [w95] mode=indexing
              n262 = xnode ("FIFO Method Node")("Element"=w95, "Timeout"=-1) -> ()  [unwired: 1 in, 2 out]
            }
          }
        }
        n263 = local read "signalToStop"() -> (w84:bool)
      }
      n264 = while {
        tunnel: "XY Clock (uSec)" -> [w327]
        stop <- w324 stop-if-true
        n265 = call "Wait"("Count(uSec)"=w327) -> ()  [unwired: 1 out]
        n266 = local read "stageIndicator"() -> (w319:u8)
        n267 = local read "x control"() -> (w321:T3)
        n268 = local read "y control"() -> (w320:T3)
        n269 = Unbundle(w321) -> ("scanning I"=w316:fxp<+,21,13>, "scanning P"=w315:fxp<+,15,5>, "Initial I (V)"=w310:fxp<+/-,10,5>, "Upper Limit (V)"=w308:fxp<+/-,26,5>, "Lower Limit (V)"=w309:fxp<+/-,26,5>, "move I"=w314:fxp<+,21,13>, "move P"=w313:fxp<+,15,5>)  [unwired: 1 out]
        n270 = Equal?(x=w319, y=u8 4) -> (x = y?=w317:bool)
        n271 = Unbundle(w320) -> ("scanning I"=w305:fxp<+,21,13>, "scanning P"=w304:fxp<+,15,5>, "Initial I (V)"=w303:fxp<+/-,10,5>, "Upper Limit (V)"=w302:fxp<+/-,26,5>, "Lower Limit (V)"=w301:fxp<+/-,26,5>, "move I"=w307:fxp<+,21,13>, "move P"=w306:fxp<+,15,5>)  [unwired: 1 out]
        n272 = Select(t=w316, s=w317, f=w314) -> (s? t:f=w312:fxp<+,21,13>)
        n273 = Select(t=w315, s=w317, f=w313) -> (s? t:f=w311:fxp<+,15,5>)
        n274 = Select(t=w305, s=w317, f=w307) -> (s? t:f=w300:fxp<+,21,13>)
        n275 = Select(t=w304, s=w317, f=w306) -> (s? t:f=w299:fxp<+,15,5>)
        n276 = xnode "FPGA I/O Node"() -> ("Mod1/AI0"=w328:fxp<+/-,20,5>)  [unwired: 1 in, 1 out]
        "x sensor" <- w328
        n277 = xnode "FPGA I/O Node"() -> ("Mod1/AI1"=w330:fxp<+/-,20,5>)  [unwired: 1 in, 1 out]
        "y sensor" <- w330
        n278 = local read "x_pos"() -> (w325:fxp<+/-,50,5>)
        n279 = local read "y_pos"() -> (w326:fxp<+/-,50,5>)
        n280 = call "PI control (SubVI).vi"("SetPoint"=w325, "Feedback"=w328, "Clock"=w327, "I"=w312, "P"=w311, "Initial I"=w310, "Lower Limit"=w309, "Upper Limit in"=w308) -> ("Output"=w323:fxp<+/-,20,5>)  [unwired: 7 in]
        "x output" <- w323
        n281 = call "PI control (SubVI).vi"("SetPoint"=w326, "Feedback"=w330, "Clock"=w327, "I"=w300, "P"=w299, "Initial I"=w303, "Lower Limit"=w301, "Upper Limit in"=w302) -> ("Output"=w329:fxp<+/-,20,5>)  [unwired: 7 in]
        "y output" <- w329
        n282 = Negate(x=w323) -> (-x=w322:fxp<+/-,21,6>)
        n283 = xnode "FPGA I/O Node"("Mod8/AO0"=w322) -> ()  [unwired: 1 in, 1 out]
        n284 = xnode "FPGA I/O Node"("Mod8/AO1"=w329) -> ()  [unwired: 1 in, 1 out]
        n285 = local read "signalToStop"() -> (w324:bool)
      }
      n286 = while {
        tunnel: "Z Clock (uSec)" -> [w264]
        stop <- w272 stop-if-true
        n287 = local read "zControlMode"() -> (w271:bool)
        n288 = call "Wait2"("Count(uSec)"=w264) -> ()  [unwired: 1 out]
        n289 = case shown="True" w271 {
          tunnel: [w280 w297] -> w270
          tunnel: [w279 w294] -> w269
          tunnel: [w275 w285] -> w268
          tunnel: [w276 w282] -> w267
          tunnel: [w278 w293] -> w266
          tunnel: [w277 w292] -> w265
          tunnel: [w274 w291] -> w263
          frame False {
            n290 = xnode "FPGA I/O Node"() -> ("Mod1/AI2"=w280:fxp<+/-,20,5>)  [unwired: 1 in, 1 out]
            n291 = local read "z control"() -> (w281:T2)
            n292 = Unbundle(w281) -> ("SetPoint (V)"=w279:fxp<+/-,26,5>, "I"=w275:fxp<+,21,13>, "P"=w276:fxp<+,15,5>, "Initial I (V)"=w274:fxp<+/-,10,5>, "Upper Limit (V)"=w277:fxp<+/-,26,5>, "Lower Limit (V)"=w278:fxp<+/-,26,5>)
          }
          frame True {
            n293 = local read "deflection control"() -> (w296:T1)
            n294 = local read "stageIndicator"() -> (w290:u8)
            n295 = xnode "FPGA I/O Node"() -> ("Mod1/AI3"=w298:fxp<+/-,20,5>)  [unwired: 1 in, 1 out]
            n296 = Equal?(x=w290, y=u8 4) -> (x = y?=w288:bool)
            n297 = Unbundle(w296) -> ("SetPoint (V)"=w295:fxp<+/-,26,5>, "scanning I"=w287:fxp<+,21,13>, "scanning P"=w284:fxp<+,15,5>, "Initial I (V)"=w291:fxp<+/-,10,5>, "Upper Limit (V)"=w292:fxp<+/-,26,5>, "Lower Limit (V)"=w293:fxp<+/-,26,5>, "approach I"=w286:fxp<+,21,13>, "approach P"=w283:fxp<+,15,5>)
            n298 = Negate(x=w298) -> (-x=w297:fxp<+/-,21,6>)
            n299 = Select(t=w287, s=w288, f=w286) -> (s? t:f=w285:fxp<+,21,13>)
            n300 = Select(t=w284, s=w288, f=w283) -> (s? t:f=w282:fxp<+,15,5>)
            n301 = Negate(x=w295) -> (-x=w294:fxp<+/-,27,6>)
          }
        }
        "deflection sensor" <- w270
        n302 = call "PI control (SubVI).vi"("SetPoint"=w269, "Feedback"=w270, "Clock"=w264, "I"=w268, "P"=w267, "Initial I"=w263, "Lower Limit"=w266, "Upper Limit in"=w265) -> ("Output"=w273:fxp<+/-,20,5>)  [unwired: 7 in]
        "z output" <- w273
        n303 = xnode "FPGA I/O Node"("Mod8/AO2"=w273) -> ()  [unwired: 1 in, 1 out]
        n304 = local read "signalToStop"() -> (w272:bool)
      }
    }
  }
